vi "CustomPID Lift.vi"(0 "Kp":dbl, 1 "Process Variable":dbl, 2 "Goal":dbl, 5 "Ki":dbl, 7 "Kd":dbl, 9 "N-Diff":i32=3, 11 "N-Int":i32=12, 12 "Reinit":bool, 13 "Max Ouput":dbl=1.0, 14 "Min Output":dbl=-1.0) -> (4 "Current Error":dbl, 8 "Command":dbl, 15 "PID Tracking":T1(graph))   [LabVIEW 2017]
uses:
  <vilib>/Analysis/NI_AALPro.lvlib
panel:
  out "x-y":u32
  out "Absolute Iterations":i32
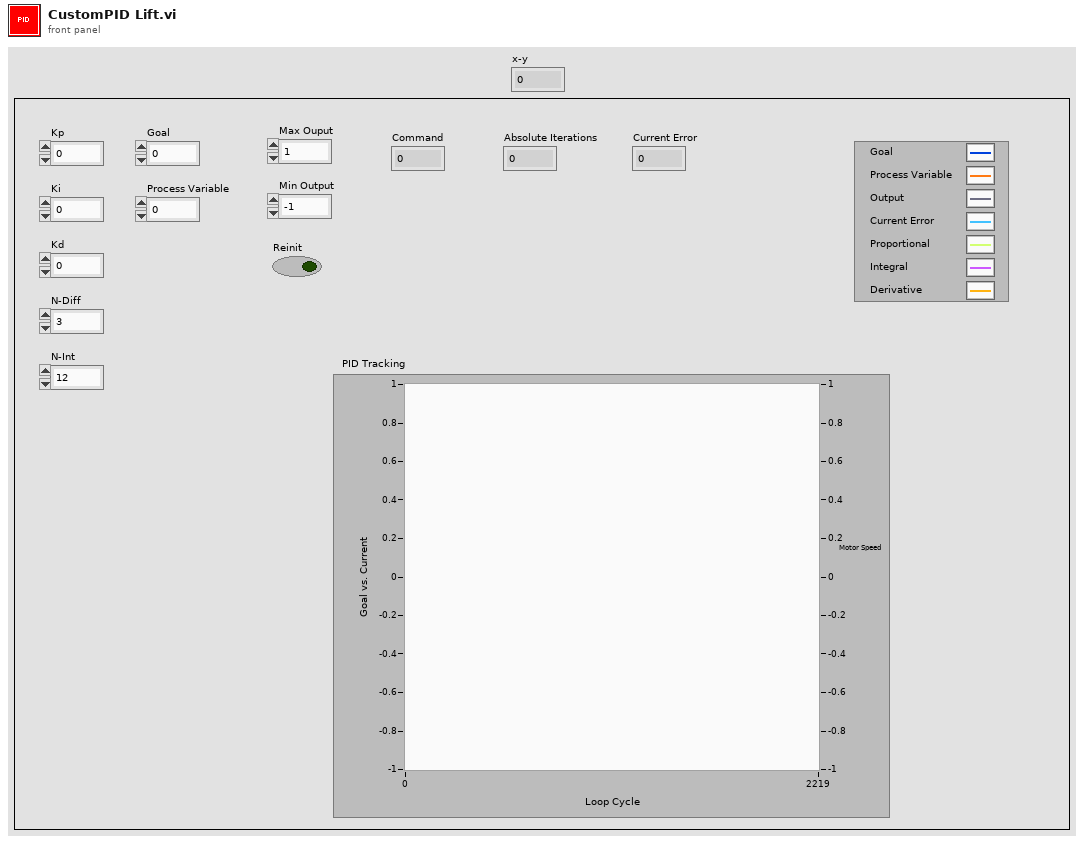
[diagram p1: front panel]
types:
  T1 = cluster{"Goal":dbl, "Process Variable":dbl, "Max Ouput":dbl, dbl, dbl, dbl, dbl}
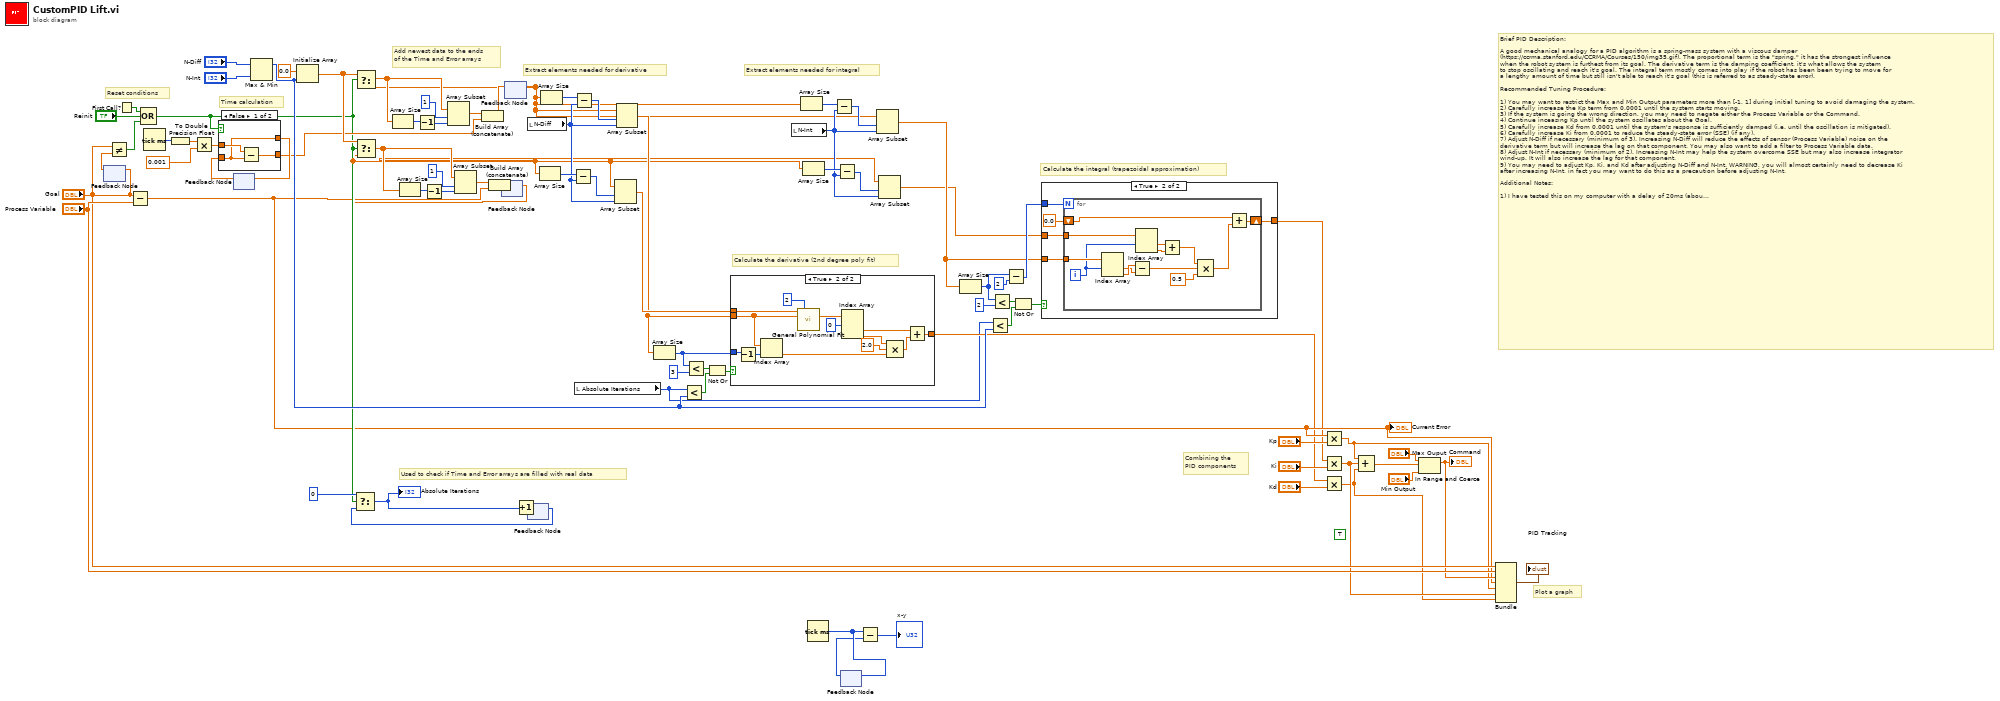
[diagram p0: block diagram]
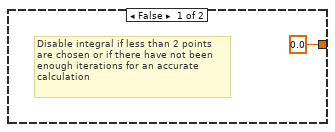
[diagram p2: hidden frame]
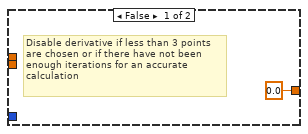
[diagram p3: hidden frame]
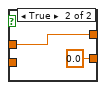
[diagram p4: hidden frame]
diagram:
  (unwired) TRUE
  # "Combining the\nPID components"
  # "Add newest data to the ends\nof the Time and Error arrays"
  # "Used to check if Time and Error arrays are filled with real data"
  # "Extract elements needed for integral"
  # "Extract elements needed for derivative"
  # "Calculate the integral (trapezoidal approximation)"
  # "Calculate the derivative (2nd degree poly fit)"
  # "Time calculation"
  # "Brief PID Description:\n\nA good mechanical analogy for a PID algorithm is a spring-mass system with a viscous damper \n(https://ccrma.stanford.edu/CCRMA/Courses/150/img35.gif). The proportional term is the \"spring,\" it has the strongest influence\nwhen the robot system is furthest from its goal. The derivative term is the damping coefficient, it's what allows the system\nto stop oscillating and reach it's goal. The integral term mostly comes into play if the robot has been been trying to move for \na lengthy amount of time but still isn't able to reach it's goal (this is referred to as steady-state error).\n\nRecommended Tuning Procedure:\n\n1) You may want to restrict the Max and Min Output parameters more than [-1, 1] during initial tuning to avoid damaging the system.\n2) Carefully increase the Kp term from 0.0001 until the system starts moving.\n3) If the system is going the wrong direction, you may need to negate either the Process Variable or the Command.\n4) Continue inceasing Kp until the system oscillates about the Goal.\n5) Carefully increase Kd from 0.0001 until the system's response is sufficiently damped (i.e. until the oscillation is mitigated).\n6) Carefully increase Ki from 0.0001 to reduce the steady-state error (SSE) (if any).\n7) Adjust N-Diff if necessary (minimum of 3). Increasing N-Diff will reduce the effects of sensor (Process Variable) noise on the \nderivative term but will increase the lag on that component. You may also want to add a filter to Process Variable data.\n8) Adjust N-Int if necessary (minimum of 2). Increasing N-Int may help the system overcome SSE but may also increase integrator\nwind-up. It will also increase the lag for that component.\n9) You may need to adjust Kp, Ki, and Kd after adjusting N-Diff and N-Int. WARNING, you will almost certainly need to decrease Ki\nafter increasing N-Int, in fact you may want to do this as a precaution before adjusting N-Int. \n\nAdditional Notes:\n\n1) I have tested this on my computer with a delay of 20ms (about what I expect for the robot) and it appears to function correctly.\nThat being said I have NOT tested this on an actual, physical system. So exercise caution when testing it for the first time.\n2) Make sure that execution type for all instances of this VI are set to \"preallocated clone reentrant execution.\"\n3) Several parts of this VI were inspired by a PID algorithm written by Dr. Ira Hill at the University of Florida.\n4) If you have any questions, feel free to contact me at lrscime@ufl.edu."
  # "Plot a graph"
  # "Reset conditions"
  n1 = feedback-in #1("Goal") -> ()
  n2 = feedback #1() -> (w69:dbl)  [unwired: 1 in]
  n3 = Not Equal?(x="Goal", y=w69) -> (x != y?=w68:bool)
  n4 = First Call?() -> (First Call?: T/F=w77:bool)
  n5 = Subtract(x="Goal", y="Process Variable") -> (x-y=w56:dbl)
  "Current Error" <- w56
  n6 = Compound Arithmetic op=OR(w77, "Reinit", w68) -> (w59:bool)
  n7 = Tick Count (ms)() -> (millisecond timer value=w66:u32)
  n8 = To Double Precision Float(number=w66) -> (double precision float=w65:dbl)
  n9 = Multiply(x=w65, y=0.001) -> (x*y=w63:dbl)
  n10 = feedback #2() -> (w61:dbl)  [unwired: 1 in]
  n11 = case shown="False" w59 {
    tunnel: w63 -> [w84 w86]
    tunnel: [w82 w86] -> w62
    tunnel: [w83 0.0] -> w60
    tunnel: w61 -> [w82 _]
    frame False {
      n12 = Subtract(x=w84, y=w82) -> (x-y=w83:dbl)
    }
    frame True {
    }
  }
  n13 = feedback-in #2(w62) -> ()
  n14 = Max & Min(x="N-Diff", y="N-Int") -> (max(x,y)=w71:i32)  [unwired: 1 out]
  n15 = Initialize Array(0.0 ("element"), w71) -> (w73:dbl[])
  n16 = feedback #3() -> (w1:dbl[])  [unwired: 1 in]
  n17 = Select(t=w73, s=w59, f=w1) -> (s? t:f=w12:dbl[])
  n18 = Array Size(array=w12) -> (size(s)=w41:i32)
  n19 = Decrement(x=w41) -> (x-1=w40:i32)
  n20 = Array Subset(array=w12, index=1, length=w40) -> (w39:dbl[])
  n21 = Build Array (concatenate)(w39, w56) -> (w2:dbl[])
  n22 = feedback-in #3(w2) -> ()
  n23 = feedback #4() -> (w3:dbl[])  [unwired: 1 in]
  n24 = Select(t=w73, s=w59, f=w3) -> (s? t:f=w13:dbl[])
  n25 = Array Size(array=w13) -> (size(s)=w45:i32)
  n26 = Decrement(x=w45) -> (x-1=w44:i32)
  n27 = Array Subset(array=w13, index=1, length=w44) -> (w43:dbl[])
  n28 = Build Array (concatenate)(w43, w60) -> (w4:dbl[])
  n29 = feedback-in #4(w4) -> ()
  n30 = local read "N-Diff"() -> (w9:i32)
  n31 = feedback #5() -> (w5:i32)  [unwired: 1 in]
  n32 = Select(t=0, s=w59, f=w5) -> (s? t:f=w11:i32)
  "Absolute Iterations" <- w11
  n33 = Increment(x=w11) -> (x+1=w6:i32)
  n34 = feedback-in #5(w6) -> ()
  n35 = Array Size(array=w1) -> (size(s)=w35:i32)
  n36 = Array Size(array=w3) -> (size(s)=w38:i32)
  n37 = Subtract(x=w35, y=w9) -> (x-y=w36:i32)
  n38 = Subtract(x=w38, y=w9) -> (x-y=w37:i32)
  n39 = local read "Absolute Iterations"() -> (w7:i32)
  n40 = Array Subset(array=w1, index=w36, length=w9) -> (w34:dbl[])
  n41 = Array Subset(array=w3, index=w37, length=w9) -> (w33:dbl[])
  n42 = Array Size(array=w33) -> (size(s)=w31:i32)
  n43 = Less?(x=w7, y=w71) -> (x < y?=w29:bool)
  n44 = Less?(x=w31, y=3) -> (x < y?=w32:bool)
  n45 = Not Or(1:w29, 2:w32) -> (0:w28:bool)
  n46 = case shown="True" w28 {
    tunnel: w34 -> [_ w93]
    tunnel: w31 -> [_ w92]
    tunnel: w33 -> [_ w90]
    tunnel: [0.0 w88] -> w27
    frame False {
      # "Disable derivative if less than 3 points \nare chosen or if there have not been \nenough iterations for an accurate \ncalculation"
    }
    frame True {
      n47 = Decrement(x=w92) -> (x-1=w91:i32)
      n48 = Index Array(array=w90, index=w91) -> (element=w89:dbl)
      n49 = call <vilib>:"General Polynomial Fit.vi"("Y"=w93, "polynomial order"=2, "X"=w90) -> ("Polynomial Coefficients"=w99:dbl[])  [unwired: 9 in, 3 out]
      n50 = Index Array(array=w99, index #1=0 ("index")) -> (element #2=w95:dbl, element #3=w97:dbl)  [unwired: 2 in, 1 out]
      n51 = Compound Arithmetic op=MULTIPLY(w97, 2.0 ("y"), w89) -> (w94:dbl)
      n52 = Add(x=w95, y=w94) -> (x+y=w88:dbl)
    }
  }
  n53 = local read "N-Int"() -> (w8:i32)
  n54 = Array Size(array=w3) -> (size(s)=w26:i32)
  n55 = Array Size(array=w1) -> (size(s)=w24:i32)
  n56 = Tick Count (ms)() -> (millisecond timer value=w52:u32)
  n57 = Subtract(x=w26, y=w8) -> (x-y=w25:i32)
  n58 = Subtract(x=w24, y=w8) -> (x-y=w23:i32)
  n59 = feedback-in #6(w52) -> ()
  n60 = feedback #6() -> (w51:u32)  [unwired: 1 in]
  n61 = Subtract(x=w52, y=w51) -> (x-y=→"x-y":u32)
  n62 = Array Subset(array=w3, index=w25, length=w8) -> (w14:dbl[])
  n63 = Array Subset(array=w1, index=w23, length=w8) -> (w10:dbl[])
  n64 = Array Size(array=w14) -> (size(s)=w17:i32)
  n65 = Less?(x=w7, y=w71) -> (x < y?=w20:bool)
  n66 = Less?(x=w17, y=2) -> (x < y?=w22:bool)
  n67 = Subtract(x=w17, y=2) -> (x-y=w16:i32)
  n68 = Not Or(1:w20, 2:w22) -> (0:w19:bool)
  n69 = case shown="True" w19 {
    tunnel: [0.0 w104] -> w18
    tunnel: w16 -> [_ w106]
    tunnel: w14 -> [_ w103]
    tunnel: w10 -> [_ w102]
    frame False {
      # "Disable integral if less than 2 points \nare chosen or if there have not been \nenough iterations for an accurate \ncalculation"
    }
    frame True {
      n70 = for {
        N: w106 -> [_]
        shift-right: [w118] -> w104
        shift-left: 0.0 -> [w119]
        tunnel: w103 -> [w117]
        tunnel: w102 -> [w110]
        i -> [w111]
        n71 = Index Array(array=w117, index #1=w111) -> (element #1=w115:dbl, element #2=w116:dbl)  [unwired: 1 in]
        n72 = Subtract(x=w116, y=w115) -> (x-y=w114:dbl)
        n73 = Index Array(array=w110, index #1=w111) -> (element #1=w108:dbl, element #2=w109:dbl)  [unwired: 1 in]
        n74 = Add(x=w108, y=w109) -> (x+y=w107:dbl)
        n75 = Compound Arithmetic op=MULTIPLY(w107, w114, 0.5 ("value")) -> (w112:dbl)
        n76 = Add(x=w119, y=w112) -> (x+y=w118:dbl)
      }
    }
  }
  n77 = Multiply(x=w56, y="Kp") -> (x*y=w55:dbl)
  n78 = Multiply(x=w18, y="Ki") -> (x*y=w54:dbl)
  n79 = Multiply(x=w27, y="Kd") -> (x*y=w53:dbl)
  n80 = Compound Arithmetic op=ADD(w55, w54, w53) -> (w80:dbl)
  n81 = In Range and Coerce(upper limit="Max Ouput", x=w80, lower limit="Min Output") -> (coerced(x)=w58:dbl)  [unwired: 1 out]
  "Command" <- w58
  n82 = Bundle("Goal"="Goal", "Process Variable"="Process Variable", "Max Ouput"=w58, w56, w55, w54, w53) -> (→"PID Tracking":T1)  [unwired: 1 in]
